vi "UI_(07A)_Set_Play_State_(offline).vi"(3 "error in (no error)":errorcluster, 4 "Settings cluster in":T1={"Defaults"={"Default User"=0.0, "VISA Resource Name "=""}, "Recording and saving"={"Researcher name"="", "Name prefix"="", "Data post-processing"={"Filter type"=enum."Savitzky-Golay", "Length"=31, "Order"=3}, "Stop at"=0.0, "\"Stop at\" enabled"=FALSE, "Default save folder path"=path "", "Acquisition FPS"=enum."Max"}, "Geometry"={"Cage diameter, mm"=0, "Starting angle MIDFIELD"=0, "Starting angle BORDER"=0, "Radius, mm CENTER"=0, "Radius, mm MIDFIELD"=0, "N segments MIDFIELD"=0, "N segments BORDER"=0, "R-gap, mm"=0.0, "Bridge swap"=FALSE, "Bridge H. offset"=0.0, "Bridge V. offset"=0.0, "Twisted neck"=FALSE, "Alt. magn. orientation"=FALSE, "Sensor board size"=enum."Small"}, "IO parameters"={"IO general config."=0, "IO 1 configuration"=0, "IO 2 configuration"=0, "IO 3 configuration"=0, "IO 4 configuration"=0, "Activate ext. RS-232"=0, "IO inversion config."=0, "Sync capability"=1}, "Stimulus presets array"=[{"Event type"=0, "Dur., s"=0.0, "Stim., s"=0.0, "TTL out N"=1, "Set/Clear"=FALSE, "Stim. has been set"=FALSE}, {"Event type"=0, "Dur., s"=0.0, "Stim., s"=0.0, "TTL out N"=1, "Set/Clear"=FALSE, "Stim. has been set"=FALSE}, {"Event type"=0, "Dur., s"=0.0, "Stim., s"=0.0, "TTL out N"=1, "Set/Clear"=FALSE, "Stim. has been set"=FALSE}, {"Event type"=0, "Dur., s"=0.0, "Stim., s"=0.0, "TTL out N"=1, "Set/Clear"=FALSE, "Stim. has been set"=FALSE}, {"Event type"=0, "Dur., s"=0.0, "Stim., s"=0.0, "TTL out N"=1, "Set/Clear"=FALSE, "Stim. has been set"=FALSE}, {"Event type"=0, "Dur., s"=0.0, "Stim., s"=0.0, "TTL out N"=1, "Set/Clear"=FALSE, "Stim. has been set"=FALSE}, {"Event type"=0, "Dur., s"=0.0, "Stim., s"=0.0, "TTL out N"=1, "Set/Clear"=FALSE, "Stim. has been set"=FALSE}, {"Event type"=0, "Dur., s"=0.0, "Stim., s"=0.0, "TTL out N"=1, "Set/Clear"=FALSE, "Stim. has been set"=FALSE}, {"Event type"=0, "Dur., s"=0.0, "Stim., s"=0.0, "TTL out N"=1, "Set/Clear"=FALSE, "Stim. has been set"=FALSE}, {"Event type"=0, "Dur., s"=0.0, "Stim., s"=0.0, "TTL out N"=1, "Set/Clear"=FALSE, "Stim. has been set"=FALSE}, {"Event type"=0, "Dur., s"=0.0, "Stim., s"=0.0, "TTL out N"=1, "Set/Clear"=FALSE, "Stim. has been set"=FALSE}, {"Event type"=0, "Dur., s"=0.0, "Stim., s"=0.0, "TTL out N"=1, "Set/Clear"=FALSE, "Stim. has been set"=FALSE}, {"Event type"=0, "Dur., s"=0.0, "Stim., s"=0.0, "TTL out N"=1, "Set/Clear"=FALSE, "Stim. has been set"=FALSE}, {"Event type"=0, "Dur., s"=0.0, "Stim., s"=0.0, "TTL out N"=1, "Set/Clear"=FALSE, "Stim. has been set"=FALSE}], "Calibration parameters"={"Timing calibration sw/hw"=1.0, "True FPS"=80.0, "True frame time, s"=0.0125, "Disp. calibration info"=[]}, "Settings loaded OK"=FALSE} {"Calibration parameters"."True frame time, s" format="%.10g"; "Calibration parameters"."Disp. calibration info"."Speed, µl per ms" format="%.3g"; "Calibration parameters"."True FPS" format="%.10g"; "Calibration parameters"."Timing calibration sw/hw" format="%.10g"; "Stimulus presets array"."Event type" items=["Stay for N seconds"]; "Stimulus presets array"."TTL out N" items=["1"=1, "2"=2, "1+2"=3]; "Recording and saving"."Data post-processing"."Order" min=3 max=11 step=2; "Recording and saving"."Data post-processing"."Length" min=5 max=301 step=2; "Geometry"."Cage diameter, mm" scale=0.0..340.0}, 5 "All references in":T11) -> (0 "error out":errorcluster, 1 "Settings cluster out":T1={"Defaults"={"Default User"=0.0, "VISA Resource Name "=""}, "Recording and saving"={"Researcher name"="", "Name prefix"="", "Data post-processing"={"Filter type"=enum."Savitzky-Golay", "Length"=31, "Order"=3}, "Stop at"=0.0, "\"Stop at\" enabled"=FALSE, "Default save folder path"=path "", "Acquisition FPS"=enum."Max"}, "Geometry"={"Cage diameter, mm"=0, "Starting angle MIDFIELD"=0, "Starting angle BORDER"=0, "Radius, mm CENTER"=0, "Radius, mm MIDFIELD"=0, "N segments MIDFIELD"=0, "N segments BORDER"=0, "R-gap, mm"=0.0, "Bridge swap"=FALSE, "Bridge H. offset"=0.0, "Bridge V. offset"=0.0, "Twisted neck"=FALSE, "Alt. magn. orientation"=FALSE, "Sensor board size"=enum."Small"}, "IO parameters"={"IO general config."=0, "IO 1 configuration"=0, "IO 2 configuration"=0, "IO 3 configuration"=0, "IO 4 configuration"=0, "Activate ext. RS-232"=0, "IO inversion config."=0, "Sync capability"=1}, "Stimulus presets array"=[{"Event type"=0, "Dur., s"=0.0, "Stim., s"=0.0, "TTL out N"=1, "Set/Clear"=FALSE, "Stim. has been set"=FALSE}, {"Event type"=0, "Dur., s"=0.0, "Stim., s"=0.0, "TTL out N"=1, "Set/Clear"=FALSE, "Stim. has been set"=FALSE}, {"Event type"=0, "Dur., s"=0.0, "Stim., s"=0.0, "TTL out N"=1, "Set/Clear"=FALSE, "Stim. has been set"=FALSE}, {"Event type"=0, "Dur., s"=0.0, "Stim., s"=0.0, "TTL out N"=1, "Set/Clear"=FALSE, "Stim. has been set"=FALSE}, {"Event type"=0, "Dur., s"=0.0, "Stim., s"=0.0, "TTL out N"=1, "Set/Clear"=FALSE, "Stim. has been set"=FALSE}, {"Event type"=0, "Dur., s"=0.0, "Stim., s"=0.0, "TTL out N"=1, "Set/Clear"=FALSE, "Stim. has been set"=FALSE}, {"Event type"=0, "Dur., s"=0.0, "Stim., s"=0.0, "TTL out N"=1, "Set/Clear"=FALSE, "Stim. has been set"=FALSE}, {"Event type"=0, "Dur., s"=0.0, "Stim., s"=0.0, "TTL out N"=1, "Set/Clear"=FALSE, "Stim. has been set"=FALSE}, {"Event type"=0, "Dur., s"=0.0, "Stim., s"=0.0, "TTL out N"=1, "Set/Clear"=FALSE, "Stim. has been set"=FALSE}, {"Event type"=0, "Dur., s"=0.0, "Stim., s"=0.0, "TTL out N"=1, "Set/Clear"=FALSE, "Stim. has been set"=FALSE}, {"Event type"=0, "Dur., s"=0.0, "Stim., s"=0.0, "TTL out N"=1, "Set/Clear"=FALSE, "Stim. has been set"=FALSE}, {"Event type"=0, "Dur., s"=0.0, "Stim., s"=0.0, "TTL out N"=1, "Set/Clear"=FALSE, "Stim. has been set"=FALSE}, {"Event type"=0, "Dur., s"=0.0, "Stim., s"=0.0, "TTL out N"=1, "Set/Clear"=FALSE, "Stim. has been set"=FALSE}, {"Event type"=0, "Dur., s"=0.0, "Stim., s"=0.0, "TTL out N"=1, "Set/Clear"=FALSE, "Stim. has been set"=FALSE}], "Calibration parameters"={"Timing calibration sw/hw"=1.0, "True FPS"=80.0, "True frame time, s"=0.0125, "Disp. calibration info"=[]}, "Settings loaded OK"=FALSE} {"Calibration parameters"."True frame time, s" format="%.10g"; "Calibration parameters"."Disp. calibration info"."Speed, µl per ms" format="%.3g"; "Calibration parameters"."True FPS" format="%.10g"; "Calibration parameters"."Timing calibration sw/hw" format="%.10g"; "Stimulus presets array"."Event type" items=["Stay for N seconds"]; "Stimulus presets array"."TTL out N" items=["1"=1, "2"=2, "1+2"=3]; "Recording and saving"."Data post-processing"."Order" min=3 max=11 step=2; "Recording and saving"."Data post-processing"."Length" min=5 max=301 step=2; "Geometry"."Cage diameter, mm" scale=0.0..340.0}, 2 "All references out":T11)   [LabVIEW 2018, in "Tracker.lvlib"]
uses:
  Tracker.lvlib
  Controls/CTL_All_References.ctl
  Controls/CTL_Controls_References.ctl
  Controls/CTL_Indicators_References.ctl
  Controls/CTL_Panes_and_VIs_References.ctl
  Controls/CTL_Histogram_Properties.ctl
  <vilib>/Utility/miscctls.llb/LVRangeTypeDef.ctl
  Controls/CTL_Settings_cluster.ctl
  Controls/CTL_Filter_selector.ctl
  Controls/CTL_Acquisition_speed_selector.ctl
  Controls/CTL_Segmented_plot_parameters.ctl
  Controls/CTL_IO_params_cluster.ctl
  Controls/CTL_Single_stimulus_setting.ctl
  Controls/CTL_Calibration_parameters.ctl
  Controls/CTL_Dispenser_calibration_info.ctl
  <vilib>/Utility/error.llb/Error Cluster From Error Code.vi
  <vilib>/ErrorRing/Error Ring.xnode
panel:
  in  "Histogram initialization cluster":T9={"X Scale.Range"={"Minimum"=0.0, "Maximum"=13.0, "Increment"=1.0, "Minor Increment"=1.0, "Start"=0.0}, "Caption.Text"="Zone preference (normalized)", "X Scale.Offset and Multiplier:Multiplier"=1.0, "X Scale.Offset and Multiplier:Offset"=0.0, "X Scale.Scale Fit"=2, "X Scale.Display Format:Precision"=0, "Y Scale.Mapping Mode"=0, "Zones preference empty initialized array"=[0, 0, 0, 0, 0, 0, 0, 0, 0, 0, 0, 0, 0, 0], "Plot.Fill/Point Color"=15790320}
  out "Panes references":T14
  out "Controls references params":string[][](array[string])
  out "Indicators references params":string[][](array[string])
  out "Indicators references":T13
  out "Controls references":T12
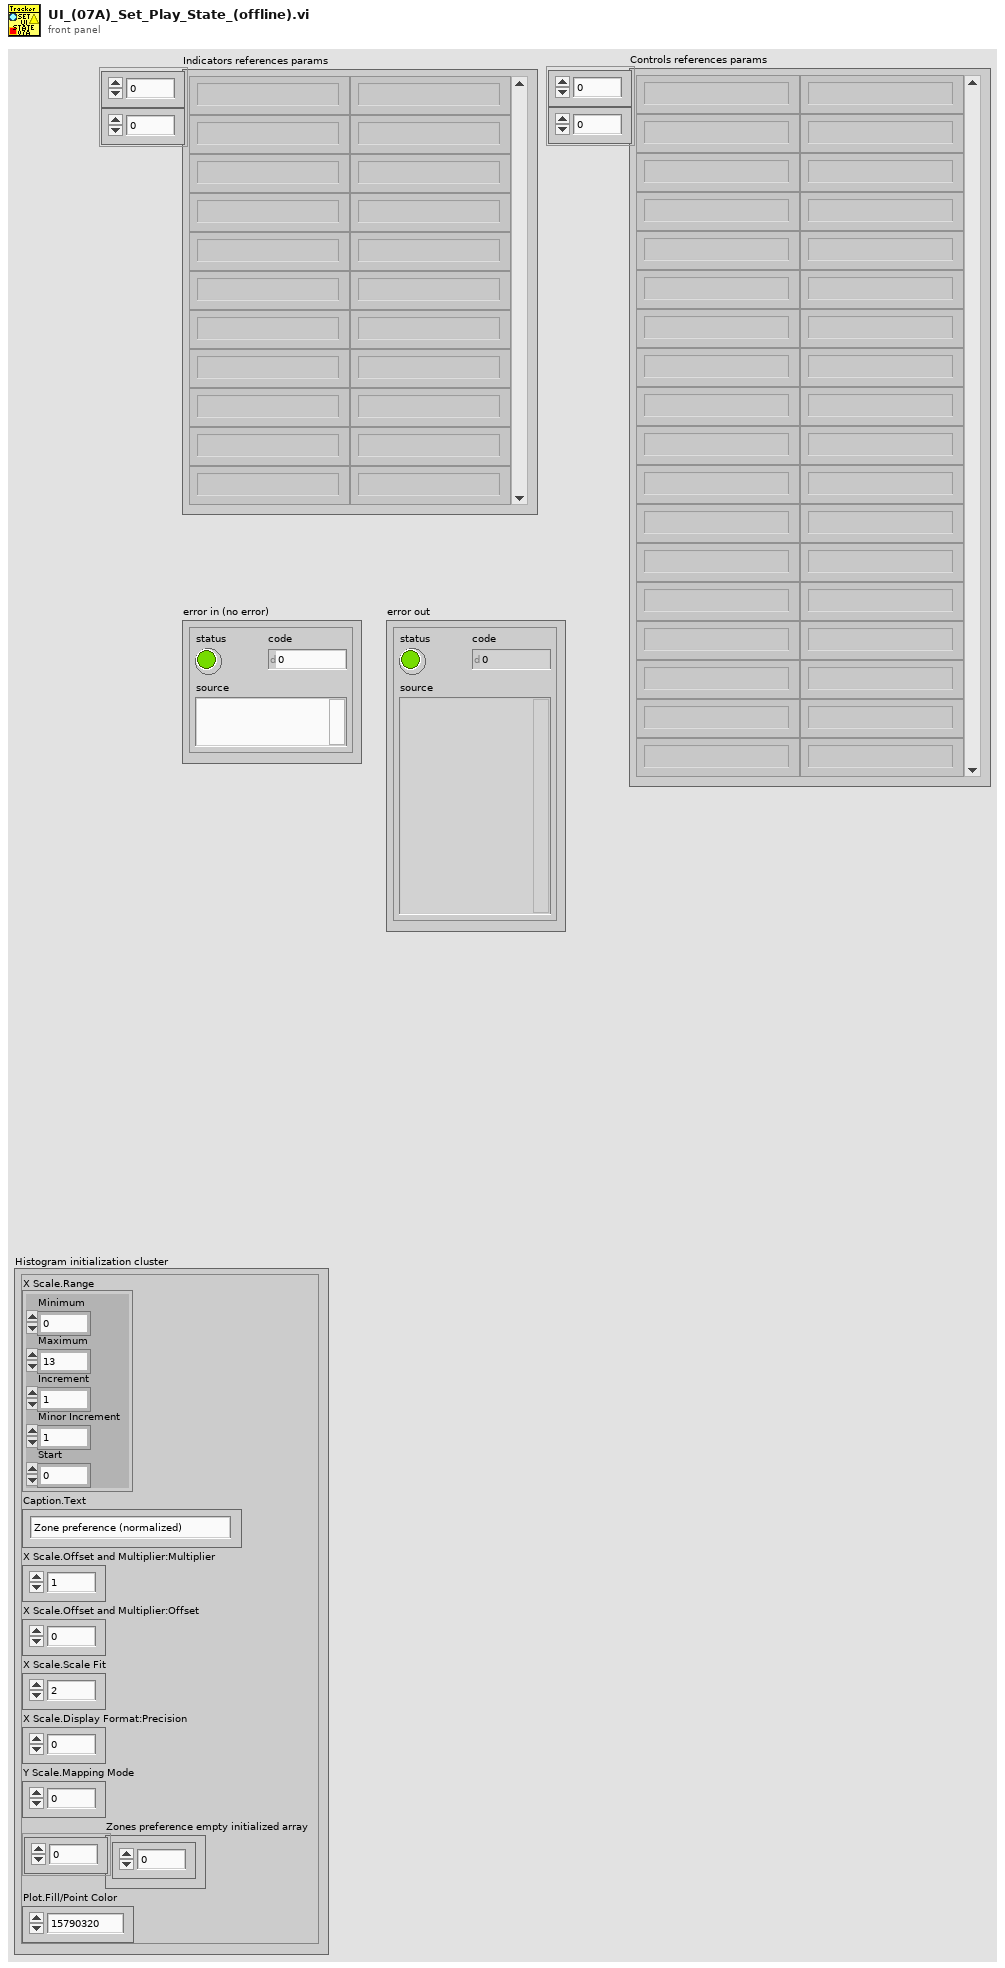
[diagram p1: front panel]
types:
  T1 = typedef "Tracker.lvlib/CTL_Settings_cluster.ctl" = cluster{"Defaults":cluster{"Default User":dbl, "VISA Resource Name ":string}, "Recording and saving":cluster{"Researcher name":string, "Name prefix":string, "Data post-processing":T2, "Stop at":dbl, "\"Stop at\" enabled":bool, "Default save folder path":path, "Acquisition FPS":T3}, "Geometry":T4, "IO parameters":T5, "Stimulus presets array":T6[], "Calibration parameters":T7, "Settings loaded OK":bool}
  T2 = typedef "Tracker.lvlib/CTL_Filter_selector.ctl" = cluster{"Filter type":enum16{"None", "Savitzky-Golay"}, "Length":i32, "Order":i32}
  T3 = typedef "Tracker.lvlib/CTL_Acquisition_speed_selector.ctl" = enum16{"Max", "Optimal", "Eco"}
  T4 = typedef "Tracker.lvlib/CTL_Segmented_plot_parameters.ctl" = cluster{"Cage diameter, mm":u16, "Starting angle MIDFIELD":i16, "Starting angle BORDER":i16, "Radius, mm CENTER":u16, "Radius, mm MIDFIELD":u16, "N segments MIDFIELD":u8, "N segments BORDER":u8, "R-gap, mm":sgl, "Bridge swap":bool, "Bridge H. offset":sgl, "Bridge V. offset":sgl, "Twisted neck":bool, "Alt. magn. orientation":bool, "Sensor board size":enum16{"Small", "Large"}}
  T5 = typedef "Tracker.lvlib/CTL_IO_params_cluster.ctl" = cluster{"IO general config.":u16, "IO 1 configuration":u16, "IO 2 configuration":u16, "IO 3 configuration":u16, "IO 4 configuration":u16, "Activate ext. RS-232":u16, "IO inversion config.":u16, "Sync capability":u8}
  T6 = typedef "Tracker.lvlib/CTL_Single_stimulus_setting.ctl" = cluster{"Event type":u16, "Dur., s":sgl, "Stim., s":sgl, "TTL out N":u16, "Set/Clear":bool, "Stim. has been set":bool}
  T7 = typedef "Tracker.lvlib/CTL_Calibration_parameters.ctl" = cluster{"Timing calibration sw/hw":dbl, "True FPS":dbl, "True frame time, s":dbl, "Disp. calibration info":T8}
  T8 = typedef "Tracker.lvlib/CTL_Dispenser_calibration_info.ctl" = cluster{"Channel":u8, "Speed, µl per ms":dbl}[]
  T9 = typedef "Tracker.lvlib/CTL_Histogram_Properties.ctl" = cluster{"X Scale.Range":T10, "Caption.Text":string, "X Scale.Offset and Multiplier:Multiplier":dbl, "X Scale.Offset and Multiplier:Offset":dbl, "X Scale.Scale Fit":u8, "X Scale.Display Format:Precision":u8, "Y Scale.Mapping Mode":u8, "Zones preference empty initialized array":i32[], "Plot.Fill/Point Color":u32}
  T10 = typedef "LVRangeTypeDef.ctl" = cluster{"Minimum":dbl, "Maximum":dbl, "Increment":dbl, "Minor Increment":dbl, "Start":dbl}
  T11 = typedef "Tracker.lvlib/CTL_All_References.ctl" = cluster{"Controls references":T12, "Indicators references":T13, "Service references":T14}
  T12 = typedef "Tracker.lvlib/CTL_Controls_References.ctl" = cluster{"Check HW connection":refnum<vi>, "Save settings":refnum<vi>, "Reset zones":refnum<vi>, "Reset stimuli":refnum<vi>, "Record/Stop":refnum<vi>, "Reset barplot":refnum<vi>, "Multiplyer of chart RX":refnum<vi>, "Show zones":refnum<vi>, "Show magnets":refnum<vi>, "Show heatmap":refnum<vi>, "Show full track":refnum<vi>, "Open File":refnum<vi>, "Play/Pause":refnum<vi>, "Trace, s":refnum<vi>, "Playback speed":refnum<vi>, "Timeline":refnum<vi>, "By Zone stim. setup":refnum<vi>, "Set/Rec and Analyse Tab":refnum<vi>, "Cage radial segmentation":refnum<vi>, "Set IO config":refnum<vi>, "Rainbow (time)":refnum<vi>, "Rainbow (speed)":refnum<vi>}
  T13 = typedef "Tracker.lvlib/CTL_Indicators_References.ctl" = cluster{"HW info":refnum<vi>, "Port":refnum<vi>, "Ready":refnum<vi>, "IO status indicator":refnum<vi>, "Current Time":refnum<vi>, "Record timestamp":refnum<vi>, "Mouse speed":refnum<vi>, "Mouse speed, mm/s":refnum<vi>, "Running, perc. of time":refnum<vi>, "Histograms":refnum<vi>, "Cage size":refnum<vi>}
  T14 = typedef "Tracker.lvlib/CTL_Panes_and_VIs_References.ctl" = cluster{"Pane":refnum<vi>, "This VI":refnum<vi>, "Menu":refnum<k9>}
  T15 = enum8{"Enabled", "Disabled", "Disabled and Grayed Out"}
  T16 = cluster{"Slider":dbl, "Slider":dbl, "Slider":dbl}
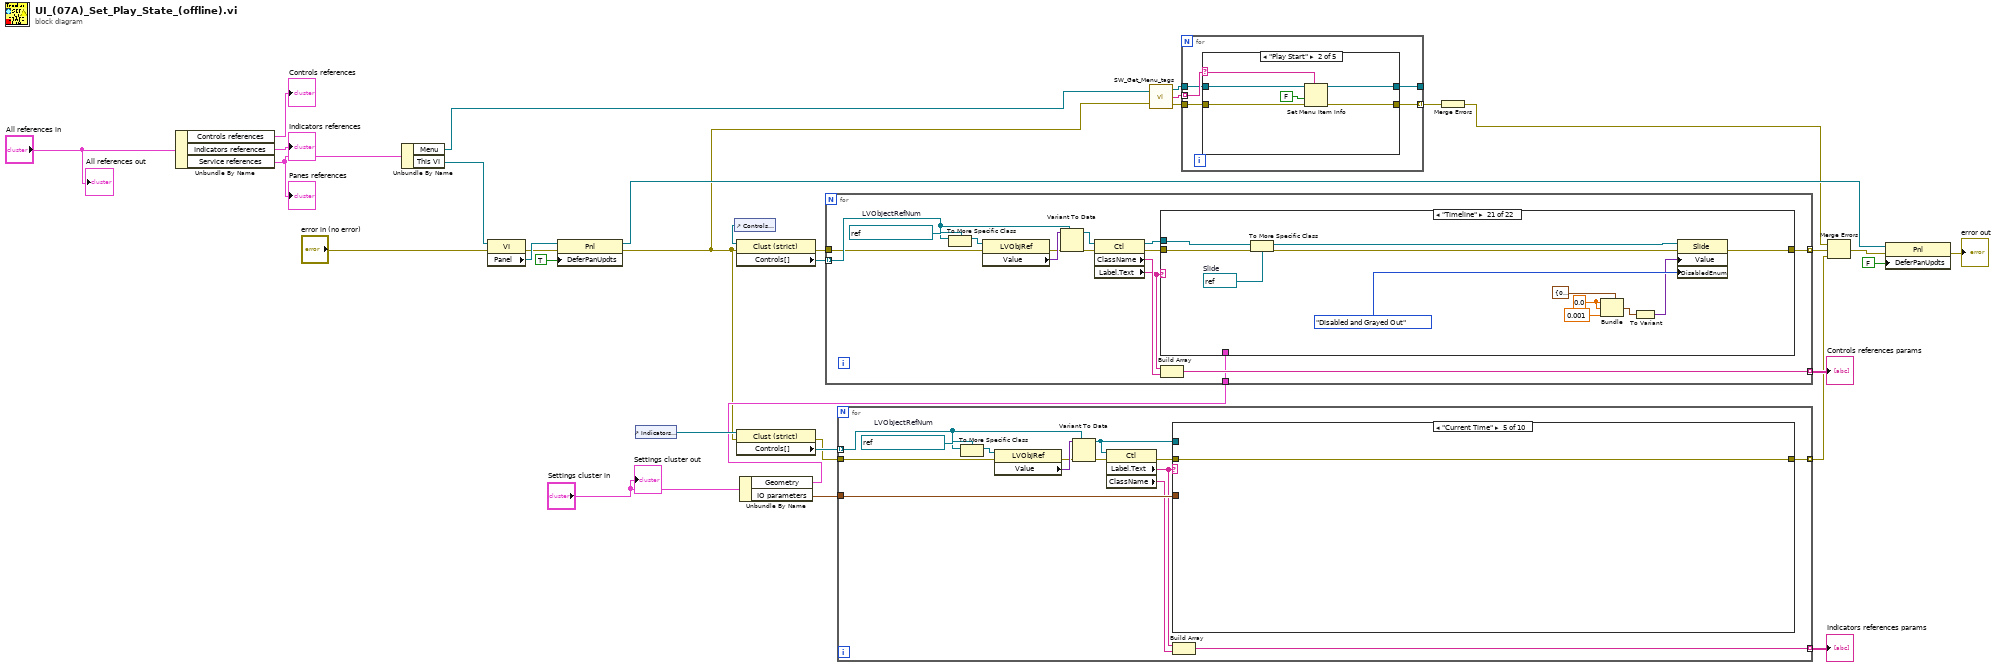
[diagram p0: block diagram]
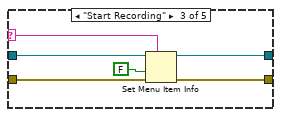
[diagram p3: hidden frame]
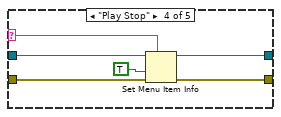
[diagram p4: hidden frame]
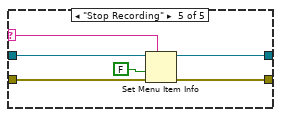
[diagram p5: hidden frame]
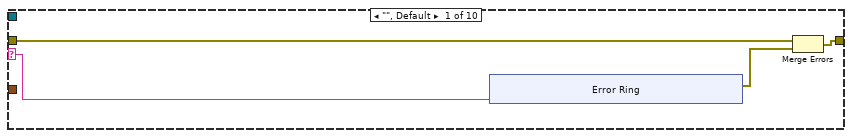
[diagram p6: hidden frame]
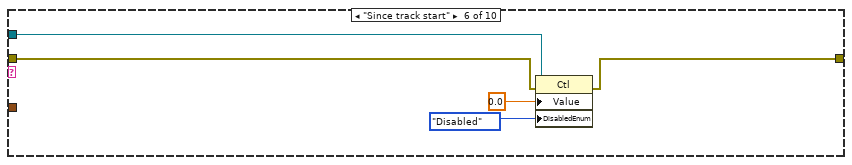
[diagram p10: hidden frame]
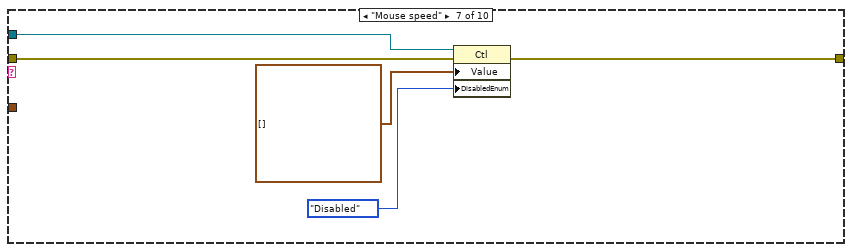
[diagram p11: hidden frame]
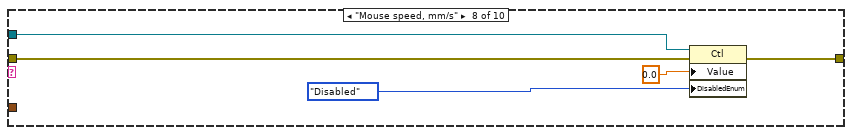
[diagram p12: hidden frame]
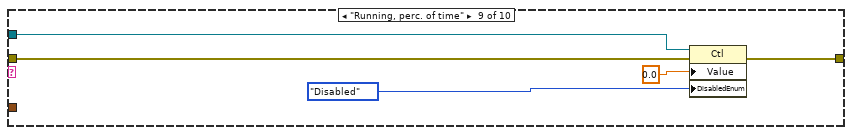
[diagram p13: hidden frame]
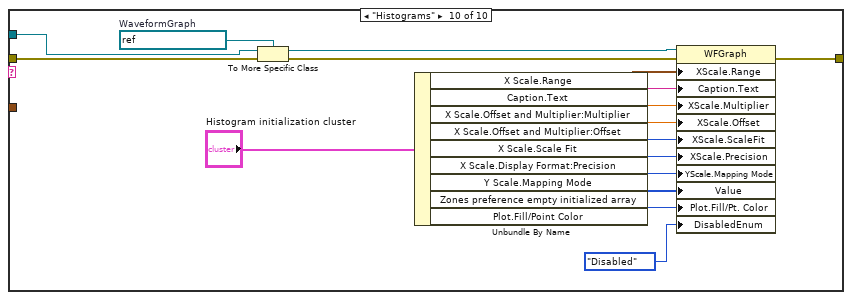
[diagram p14: hidden frame]
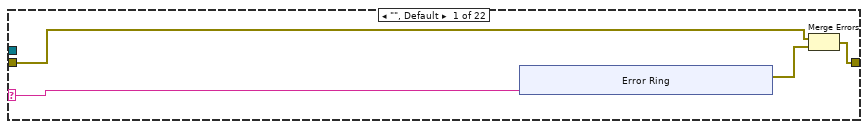
[diagram p15: hidden frame]
diagram:
  n1 = Unbundle By Name("All references in") -> ("Controls references"=→"Controls references":T12, "Indicators references"=→"Indicators references":T13, "Service references"=w24:T14)
  "Panes references" <- w24
  n2 = Unbundle By Name(w24) -> ("Menu"=w3:refnum<k9>, "This VI"=w21:refnum<vi>)
  n3 = property class="VI"(reference=w21, error in="error in (no error)") -> (error out=w14:errorcluster, "Panel"=w23:refnum<vi>)  [unwired: 1 out]
  n4 = property class="Pnl"(reference=w23, error in=w14, "DeferPanUpdts"=TRUE ("Defer Panel Updates")) -> (reference out=w15:refnum<vi>, error out=w2:errorcluster)
  n5 = control-ref of="Indicators references"() -> (w27:refnum<vi>)
  n6 = control-ref of="Controls references"() -> (w29:refnum<vi>)
  n7 = property class="Clust (strict)"(reference=w29, error in=w2) -> (error out=w20:errorcluster, "Controls[]"=w30:refnum<vi>[])  [unwired: 1 out]
  n8 = property class="Clust (strict)"(reference=w27, error in=w2) -> (error out=w19:errorcluster, "Controls[]"=w28:refnum<vi>[])  [unwired: 1 out]
  n9 = Unbundle By Name("Settings cluster in") -> ("Geometry"=w8:T4, "IO parameters"=w10:T5)
  n10 = for {
    tunnel: w30 -> [w45] mode=indexing
    tunnel: [w42] -> w25 mode=indexing
    tunnel: w20 -> [w41]
    tunnel: [w37] -> w12 mode=indexing
    tunnel: w8 -> [w34]
    w47 = refnum<vi> refnum  # LVObjectRefNum
    n11 = To More Specific Class(target class=w47, reference=w45) -> (specific class reference=w48:refnum<vi>)  [unwired: 1 in, 1 out]
    n12 = property class="LVObjRef"(reference=w48, error in=w41) -> (error out=w40:errorcluster, "Value"=w46:variant)  [unwired: 1 out]
    n13 = Variant To Data(error in=w40, type=w45, Variant=w46) -> (data=w44:refnum<vi>, error out=w39:errorcluster)
    n14 = property class="Ctl"(reference=w44, error in=w39) -> (reference out=w35:refnum<vi>, error out=w36:errorcluster, "ClassName"=w43:string, "Label.Text"=w38:string)
    n15 = case shown="\"Timeline\"" w38 {
      selector: w38 -> [w49 _ _ _ _ _ _ _ _ _ _ _ _ _ _ _ _ _ _ _ _ _]
      tunnel: [w51 w60 w61 w62 w63 w64 w65 w66 w69 w77 w85 w93 w99 w100 w109 w115 w125 w126 w129 w137 w149 w155] -> w37
      tunnel: w36 -> [w52 w60 w61 w62 w63 w64 w65 w66 w71 w79 w87 w95 w99 w102 w111 w115 w125 w126 w131 w139 w151 w155]
      tunnel: w35 -> [_ _ _ _ _ _ _ _ w74 w82 w90 w98 _ w101 w114 w116 _ _ w134 w142 w154 _]
      tunnel: w34 -> [_ _ _ _ _ _ _ _ _ _ _ _ _ _ _ _ _ _ _ _ _ _]
      frame "", Default {
        n16 = xnode "Error Ring"("parameter 0"=w49) -> ("error out"=w50:errorcluster)
        n17 = Merge Errors(w52, w50) -> (w51:errorcluster)
      }
      frame "Cage radial segmentation" {
      }
      frame "Set/Rec and Analyse Tab" {
      }
      frame "Check HW connection" {
      }
      frame "Save settings" {
      }
      frame "Set IO config" {
      }
      frame "Reset zones" {
      }
      frame "Reset stimuli" {
      }
      frame "Record/Stop" {
        w73 = refnum<vi> refnum  # Boolean
        n18 = To More Specific Class(target class=w73, reference=w74, error in=w71) -> (specific class reference=w72:refnum<vi>, error out=w70:errorcluster)
        n19 = property class="Bool"(reference=w72, error in=w70, "Value"=FALSE, "DisabledEnum"=T15."Disabled and Grayed Out" ("Disabled")) -> (error out=w69:errorcluster)  [unwired: 1 out]
      }
      frame "Reset barplot" {
        w81 = refnum<vi> refnum  # Boolean
        n20 = To More Specific Class(target class=w81, reference=w82, error in=w79) -> (specific class reference=w80:refnum<vi>, error out=w78:errorcluster)
        n21 = property class="Bool"(reference=w80, error in=w78, "Value"=FALSE, "DisabledEnum"=T15."Enabled" ("Disabled")) -> (error out=w77:errorcluster)  [unwired: 1 out]
      }
      frame "Multiplyer of chart RX" {
        w89 = refnum<vi> refnum  # Slide
        n22 = To More Specific Class(target class=w89, reference=w90, error in=w87) -> (specific class reference=w88:refnum<vi>, error out=w86:errorcluster)
        n23 = property class="Slide"(reference=w88, error in=w86, "Value"=u8 1, "DisabledEnum"=T15."Enabled" ("Disabled")) -> (error out=w85:errorcluster)  [unwired: 1 out]
      }
      frame "Show zones" {
        w97 = refnum<vi> refnum  # Boolean
        n24 = To More Specific Class(target class=w97, reference=w98, error in=w95) -> (specific class reference=w96:refnum<vi>, error out=w94:errorcluster)
        n25 = property class="Bool"(reference=w96, error in=w94, "Value"=TRUE, "DisabledEnum"=T15."Enabled" ("Disabled")) -> (error out=w93:errorcluster)  [unwired: 1 out]
      }
      frame "Show magnets" {
      }
      frame "Rainbow (speed)", "Rainbow (time)" {
        w103 = refnum<vi> refnum  # Boolean
        n26 = To More Specific Class(target class=w103, reference=w101, error in=w102) -> (specific class reference=w105:refnum<vi>, error out=w106:errorcluster)
        n27 = property class="Bool"(reference=w105, error in=w106, "DisabledEnum"=T15."Enabled" ("Disabled")) -> (error out=w100:errorcluster)  [unwired: 1 out]
      }
      frame "Show heatmap" {
        w113 = refnum<vi> refnum  # Boolean
        n28 = To More Specific Class(target class=w113, reference=w114, error in=w111) -> (specific class reference=w112:refnum<vi>, error out=w110:errorcluster)
        n29 = property class="Bool"(reference=w112, error in=w110, "Value"=FALSE, "DisabledEnum"=T15."Disabled and Grayed Out" ("Disabled")) -> (error out=w109:errorcluster)  [unwired: 1 out]
      }
      frame "Show full track" {
        n30 = disable-structure shown="Disabled" {
          disable-tunnel: w116 -> [w124 _]
          disable-tunnel: _ -> [w121 _]
          disable-tunnel: [w119 _] -> _
          frame Disabled {
            w123 = refnum<vi> refnum  # Boolean
            n31 = To More Specific Class(target class=w123, reference=w124, error in=w121) -> (specific class reference=w122:refnum<vi>, error out=w120:errorcluster)
            n32 = property class="Bool"(reference=w122, error in=w120, "Value"=FALSE, "DisabledEnum"=T15."Disabled and Grayed Out" ("Disabled")) -> (error out=w119:errorcluster)  [unwired: 1 out]
          }
          frame Enabled {
          }
        }
      }
      frame "Open File" {
      }
      frame "Play/Pause" {
      }
      frame "Trace, s" {
        w133 = refnum<vi> refnum  # Slide
        n33 = To More Specific Class(target class=w133, reference=w134, error in=w131) -> (specific class reference=w132:refnum<vi>, error out=w130:errorcluster)
        n34 = property class="Slide"(reference=w132, error in=w130, "Value"=u8 5, "DisabledEnum"=T15."Enabled" ("Disabled")) -> (error out=w129:errorcluster)  [unwired: 1 out]
      }
      frame "Playback speed" {
        w141 = refnum<vi> refnum  # Ring
        n35 = To More Specific Class(target class=w141, reference=w142, error in=w139) -> (specific class reference=w140:refnum<vi>, error out=w138:errorcluster)
        n36 = property class="Ring"(reference=w140, error in=w138, "Value"=u8 3, "DisabledEnum"=T15."Disabled and Grayed Out" ("Disabled")) -> (error out=w137:errorcluster)  [unwired: 1 out]
      }
      frame "Timeline" {
        w145 = 0.0 ("Slider")
        w153 = refnum<vi> refnum  # Slide
        n37 = To More Specific Class(target class=w153, reference=w154, error in=w151) -> (specific class reference=w152:refnum<vi>, error out=w150:errorcluster)
        n38 = Bundle(cluster=T16 {"Slider"=0.0, "Slider"=0.0, "Slider"=0.0} ("Timeline"), "Slider"=w145, "Slider"=w145, "Slider"=0.001) -> (w146:T16)
        n39 = To Variant(anything=w146) -> (Variant=w143:variant)
        n40 = property class="Slide"(reference=w152, error in=w150, "Value"=w143, "DisabledEnum"=T15."Disabled and Grayed Out" ("Disabled")) -> (error out=w149:errorcluster)  [unwired: 1 out]
      }
      frame "By Zone stim. setup" {
      }
    }
    n41 = Build Array(w38, w43) -> (w42:string[])
  }
  "Controls references params" <- w25
  n42 = for {
    tunnel: w28 -> [w166] mode=indexing
    tunnel: [w156] -> w26 mode=indexing
    tunnel: w19 -> [w164]
    tunnel: [w160] -> w18 mode=indexing
    tunnel: w10 -> [w159]
    w168 = refnum<vi> refnum  # LVObjectRefNum
    n43 = To More Specific Class(target class=w168, reference=w166) -> (specific class reference=w169:refnum<vi>)  [unwired: 1 in, 1 out]
    n44 = property class="LVObjRef"(reference=w169, error in=w164) -> (error out=w163:errorcluster, "Value"=w167:variant)  [unwired: 1 out]
    n45 = Variant To Data(error in=w163, type=w166, Variant=w167) -> (data=w165:refnum<vi>, error out=w162:errorcluster)
    n46 = property class="Ctl"(reference=w165, error in=w162) -> (error out=w161:errorcluster, "Label.Text"=w158:string, "ClassName"=w157:string)  [unwired: 1 out]
    n47 = case shown="\"Current Time\"" w158 {
      selector: w158 -> [w170 _ _ _ _ _ _ _ _ _]
      tunnel: w165 -> [_ _ _ _ _ w185 w194 w199 w204 w221]
      tunnel: w161 -> [w173 w181 w182 w183 w184 w187 w193 w198 w203 w207]
      tunnel: [w172 w181 w182 w183 w184 w186 w192 w197 w202 w220] -> w160
      tunnel: w159 -> [_ _ _ _ _ _ _ _ _ _]
      frame "", Default {
        n48 = xnode "Error Ring"("parameter 0"=w170) -> ("error out"=w171:errorcluster)
        n49 = Merge Errors(w173, w171) -> (w172:errorcluster)
      }
      frame "Cage size", "HW info", "Port" {
      }
      frame "Ready" {
      }
      frame "IO status indicator" {
      }
      frame "Current Time" {
      }
      frame "Since track start" {
        n50 = property class="Ctl"(reference=w185, error in=w187, "Value"=0.0, "DisabledEnum"=T15."Disabled" ("Disabled")) -> (error out=w186:errorcluster)  [unwired: 1 out]
      }
      frame "Mouse speed" {
        n51 = property class="Ctl"(reference=w194, error in=w193, "Value"=waveform(dbl)[] [] ("History Data"), "DisabledEnum"=T15."Disabled" ("Disabled")) -> (error out=w192:errorcluster)  [unwired: 1 out]
      }
      frame "Mouse speed, mm/s" {
        n52 = property class="Ctl"(reference=w199, error in=w198, "Value"=0.0, "DisabledEnum"=T15."Disabled" ("Disabled")) -> (error out=w197:errorcluster)  [unwired: 1 out]
      }
      frame "Running, perc. of time" {
        n53 = property class="Ctl"(reference=w204, error in=w203, "Value"=0.0, "DisabledEnum"=T15."Disabled" ("Disabled")) -> (error out=w202:errorcluster)  [unwired: 1 out]
      }
      frame "Histograms" {
        w218 = refnum<vi> refnum  # WaveformGraph
        n54 = To More Specific Class(target class=w218, reference=w221, error in=w207) -> (specific class reference=w219:refnum<vi>, error out=w206:errorcluster)
        n55 = Unbundle By Name("Histogram initialization cluster") -> ("X Scale.Range"=w216:T10, "Caption.Text"=w215:string, "X Scale.Offset and Multiplier:Multiplier"=w214:dbl, "X Scale.Offset and Multiplier:Offset"=w213:dbl, "X Scale.Scale Fit"=w212:u8, "X Scale.Display Format:Precision"=w211:u8, "Y Scale.Mapping Mode"=w210:u8, "Zones preference empty initialized array"=w209:i32[], "Plot.Fill/Point Color"=w208:u32)
        n56 = property class="WFGraph"(reference=w219, error in=w206, "XScale.Range"=w216, "Caption.Text"=w215, "XScale.Multiplier"=w214, "XScale.Offset"=w213, "XScale.ScaleFit"=w212, "XScale.Precision"=w211, "YScale.Mapping Mode"=w210, "Value"=w209, "Plot.Fill/Pt. Color"=w208, "DisabledEnum"=T15."Disabled" ("Disabled")) -> (error out=w220:errorcluster)  [unwired: 1 out]
      }
    }
    n57 = Build Array(w158, w157) -> (w156:string[])
  }
  "Indicators references params" <- w26
  n58 = call "SW_Get_Menu_tags.vi"("Menu ref in"=w3, "error in (no error)"=w2) -> ("Menu ref out"=w5:refnum<k9>, "(Sub)menu tags"=w7:string[], "error out"=w6:errorcluster)
  n59 = for {
    tunnel: w7 -> [w226] mode=indexing
    tunnel: w6 -> [w225]
    tunnel: [w224] -> w4 mode=indexing
    tunnel: [w223] -> _
    tunnel: w5 -> [w222]
    n60 = case shown="\"Play Start\"" w226 {
      selector: w226 -> [_ w234 w240 w246 w252]
      tunnel: w225 -> [w228 w232 w238 w244 w250]
      tunnel: [w228 w231 w237 w243 w249] -> w224
      tunnel: [w227 w230 w236 w242 w248] -> w223
      tunnel: w222 -> [w227 w229 w235 w241 w247]
      frame "", Default {
      }
      frame "Play Start" {
        n61 = Set Menu Item Info(7:w234, 8:w232, 9:FALSE ("enabled"), 11:w229) -> (0:w231:errorcluster, 3:w230:refnum<k9>)  [unwired: 3 in]
      }
      frame "Start Recording" {
        n62 = Set Menu Item Info(7:w240, 8:w238, 9:FALSE ("enabled"), 11:w235) -> (0:w237:errorcluster, 3:w236:refnum<k9>)  [unwired: 3 in]
      }
      frame "Play Stop" {
        n63 = Set Menu Item Info(7:w246, 8:w244, 9:TRUE ("enabled"), 11:w241) -> (0:w243:errorcluster, 3:w242:refnum<k9>)  [unwired: 3 in]
      }
      frame "Stop Recording" {
        n64 = Set Menu Item Info(7:w252, 8:w250, 9:FALSE ("enabled"), 11:w247) -> (0:w249:errorcluster, 3:w248:refnum<k9>)  [unwired: 3 in]
      }
    }
  }
  n65 = Merge Errors(w4) -> (w1:errorcluster)
  n66 = Merge Errors(w1, w12, w18) -> (w17:errorcluster)
  n67 = property class="Pnl"(reference=w15, error in=w17, "DeferPanUpdts"=FALSE ("Defer Panel Updates")) -> (error out=→"error out":errorcluster)  [unwired: 1 out]
  "All references out" <- "All references in"
  "Settings cluster out" <- "Settings cluster in"
